vi "GantryControl.vi"(8 "error in":errorcluster) -> ()   [LabVIEW 2014]
uses:
  Utilities/ButtonBoxVars.vi
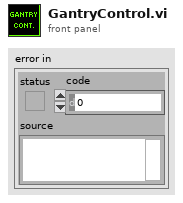
[diagram p1: front panel]
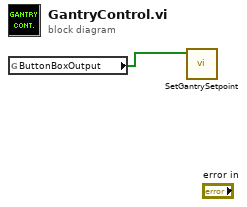
[diagram p0: block diagram]
diagram:
  n1 = global read "ButtonBoxVars.vi" "ButtonBoxOutput"() -> (w1:bool[])
  n2 = call "SetGantrySetpoint.vi"("Buttons"=w1) -> ()  [unwired: 11 in]
